vi "Save-raw-path.vi"(8 "error in (no error)":errorcluster, 11 "Reference in":T1) -> (0 "error out":errorcluster, 3 "Reference out":T1)   [LabVIEW 2013, in "MaterialCharacterization.lvlib" / "MC-ScanParser.lvclass"]
uses:
  MC-ScanParser.lvclass
  Object-reference.ctl
  MC-ScanParser.lvclass/MC-ScanParser.ctl
  Read Scan file path.vi
  <vilib>/Utility/file.llb/Write To Spreadsheet File (string).vi
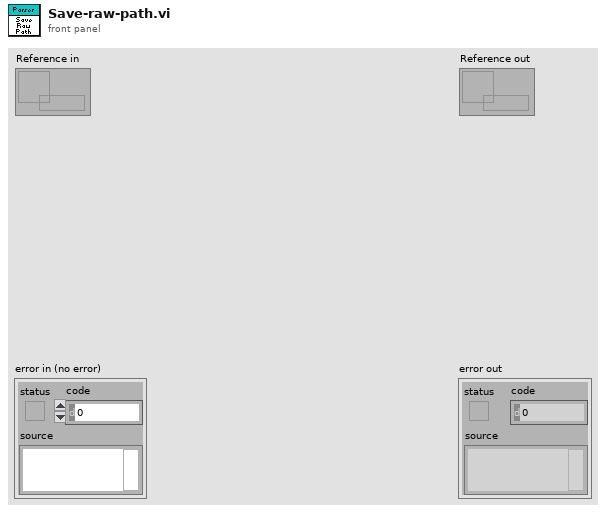
[diagram p1: front panel]
types:
  T1 = typedef "MaterialCharacterization.lvlib/MC-ScanParser.lvclass/Object-reference.ctl" = refnum<data-value>
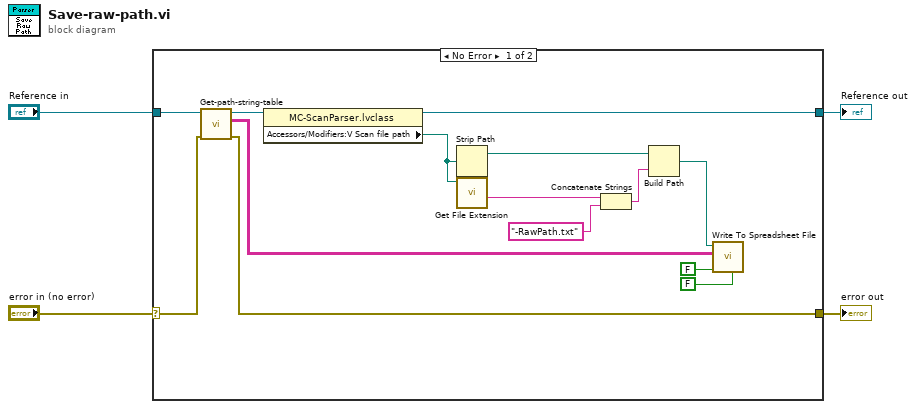
[diagram p0: block diagram]
diagram:
  n1 = case shown="No Error" "error in (no error)" {
    selector: "error in (no error)" -> [w14 w19]
    tunnel: [w9 w19] -> w3
    tunnel: [w18 w20] -> w1
    tunnel: "Reference in" -> [w15 w20]
    frame No Error {
      n2 = call "Get-path-string-table.vi"("error in (no error)"=w14, "Reference in"=w15) -> ("error out"=w9:errorcluster, "String table"=w13:string[][], "Reference out"=w8:T1)  [unwired: 7 in]
      n3 = property class="MC-ScanParser.lvclass"(reference=w8) -> (reference out=w18:T1, "Accessors/Modifiers:V Scan file path"=w7:path)  [unwired: 1 in, 1 out]
      n4 = Strip Path(path=w7) -> (stripped path=w17:path)  [unwired: 1 out]
      n5 = call <vilib>:"Get File Extension.vi"("file"=w7) -> ("filename without extension"=w6:string)  [unwired: 7 in, 3 out]
      n6 = Concatenate Strings(w6, "-RawPath.txt" ("string")) -> (w16:string)
      n7 = Build Path(base path=w17, name or relative path=w16) -> (appended path=w12:path)
      n8 = call-poly <vilib>:"Write To Spreadsheet File.vi"("transpose? (no:F)"=FALSE, "append to file? (new file:F)"=FALSE, "2D data"=w13, "file path (dialog if empty)"=w12) -> ()  [unwired: 4 in, 1 out]
    }
    frame Error {
    }
  }
  "error out" <- w3
  "Reference out" <- w1
